vi "CondDoubleArrayProbe.vi"(1 "My Array In":dbl[](array[numeric])) -> (0 "Boolean":bool)   [LabVIEW 2020]
doc: "Monitors an array of double-precision, floating-point numeric controls. The Data tab displays the size of the input array. Use the Conditions tab to set a conditional breakpoint. You can set conditions based on the size of the array or any elements within the array. If you select multiple conditions, LabVIEW executes a breakpoint if any of those conditions are true."
panel:
  in  "Tab Control":enum32{"Data   ", "Conditions      "}(tab)
  out "?":dbl[](array[numeric])
  out "Size of array":i32
  in  "Max Condition":u16(ring) items=["Equal to", "Greater than", "Less than"]
  in  "Max value":dbl
  in  "Maximum value is":bool
  in  "Min Condition":u16(ring) items=["Equal to", "Greater than", "Less than"]
  in  "Min value":dbl
  in  "Minimum value is":bool
  in  "Contains Condition":u16(ring) items=["Equal to", "Greater than", "Less than"]
  in  "Contains value":dbl
  in  "Contains a value":bool
  in  "Number of \nElements Condition":u16(ring) items=["Equal to", "Greater than", "Less than"]
  in  "Number of \nelements value":u32
  in  "Number of \nelements is":bool
  # "Pause if any of the following:"
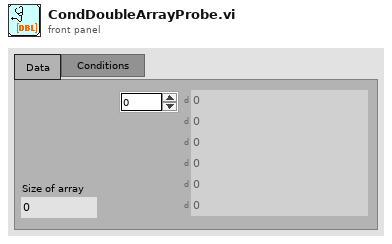
[diagram p1: front panel]
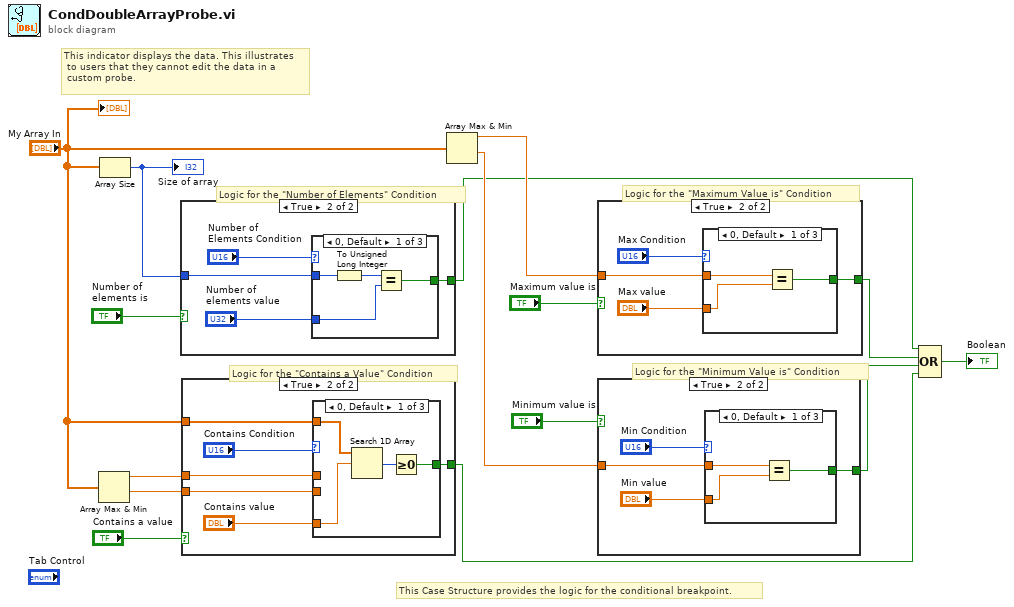
[diagram p0: block diagram]
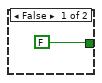
[diagram p2: hidden frame]
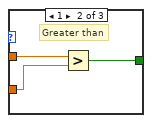
[diagram p3: hidden frame]
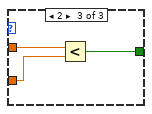
[diagram p4: hidden frame]
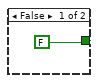
[diagram p5: hidden frame]
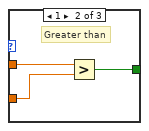
[diagram p6: hidden frame]
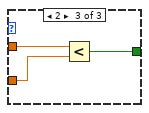
[diagram p7: hidden frame]
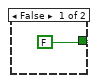
[diagram p8: hidden frame]
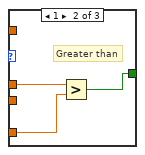
[diagram p9: hidden frame]
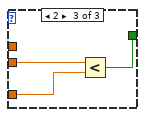
[diagram p10: hidden frame]
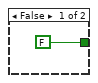
[diagram p11: hidden frame]
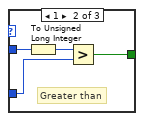
[diagram p12: hidden frame]
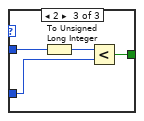
[diagram p13: hidden frame]
diagram:
  # "This indicator displays the data. This illustrates\n to users that they cannot edit the data in a\n custom probe."
  # "Logic for the \"Maximum Value is\" Condition"
  # "Logic for the \"Minimum Value is\" Condition"
  # "Logic for the \"Contains a Value\" Condition"
  # "Logic for the \"Number of Elements\" Condition"
  # "This Case Structure provides the logic for the conditional breakpoint."
  n1 = Array Max & Min(array="My Array In") -> (max value=w12:dbl, min value=w13:dbl)  [unwired: 2 out]
  n2 = Array Size(array="My Array In") -> (size(s)=w14:i32)
  "Size of array" <- w14
  n3 = case shown="True" "Number of \nelements is" {
    tunnel: w14 -> [_ w19]
    tunnel: [FALSE w17] -> w1
    frame False {
    }
    frame True {
      n4 = case shown="0, Default" "Number of \nElements Condition" {
        tunnel: [w24 w26 w30] -> w17
        tunnel: w19 -> [w23 w28 w32]
        tunnel: "Number of \nelements value" -> [w22 w27 w31]
        frame 0, Default {
          n5 = To Unsigned Long Integer(number=w23) -> (unsigned 32bit integer=w21:u32)
          n6 = Equal?(x=w21, y=w22) -> (x = y?=w24:bool)
        }
        frame 1 {
          # "Greater than"
          n7 = To Unsigned Long Integer(number=w28) -> (unsigned 32bit integer=w25:u32)
          n8 = Greater?(x=w25, y=w27) -> (0:w26:bool)
        }
        frame 2 {
          n9 = To Unsigned Long Integer(number=w32) -> (unsigned 32bit integer=w29:u32)
          n10 = Less?(x=w29, y=w31) -> (x < y?=w30:bool)
        }
      }
    }
  }
  n11 = case shown="True" "Contains a value" {
    tunnel: "My Array In" -> [_ w38]
    tunnel: [FALSE w35] -> w5
    tunnel: w12 -> [_ w37]
    tunnel: w13 -> [_ w36]
    frame False {
    }
    frame True {
      n12 = case shown="0, Default" "Contains Condition" {
        tunnel: [w40 w46 w49] -> w35
        tunnel: "Contains value" -> [w42 w44 w48]
        tunnel: w38 -> [w41 _ _]
        tunnel: w37 -> [_ w45 _]
        tunnel: w36 -> [_ _ w47]
        frame 0, Default {
          n13 = Search 1D Array(1D array=w41, element=w42) -> (index of element=w43:i32)  [unwired: 1 in]
          n14 = Greater Or Equal To 0?(x=w43) -> (x >= 0?=w40:bool)
        }
        frame 1 {
          # "Greater than"
          n15 = Greater?(x=w45, y=w44) -> (0:w46:bool)
        }
        frame 2 {
          n16 = Less?(x=w47, y=w48) -> (x < y?=w49:bool)
        }
      }
    }
  }
  n17 = Array Max & Min(array="My Array In") -> (max value=w8:dbl, min value=w7:dbl)  [unwired: 2 out]
  n18 = case shown="True" "Maximum value is" {
    tunnel: [FALSE w52] -> w2
    tunnel: w8 -> [_ w53]
    frame False {
    }
    frame True {
      n19 = case shown="0, Default" "Max Condition" {
        tunnel: [w57 w58 w61] -> w52
        tunnel: w53 -> [w56 w60 w63]
        tunnel: "Max value" -> [w55 w59 w62]
        frame 0, Default {
          n20 = Equal?(x=w56, y=w55) -> (x = y?=w57:bool)
        }
        frame 1 {
          # "Greater than"
          n21 = Greater?(x=w60, y=w59) -> (0:w58:bool)
        }
        frame 2 {
          n22 = Less?(x=w63, y=w62) -> (x < y?=w61:bool)
        }
      }
    }
  }
  n23 = case shown="True" "Minimum value is" {
    tunnel: w7 -> [_ w66]
    tunnel: [FALSE w65] -> w3
    frame False {
    }
    frame True {
      n24 = case shown="0, Default" "Min Condition" {
        tunnel: [w71 w72 w75] -> w65
        tunnel: w66 -> [w70 w74 w77]
        tunnel: "Min value" -> [w69 w73 w76]
        frame 0, Default {
          n25 = Equal?(x=w70, y=w69) -> (x = y?=w71:bool)
        }
        frame 1 {
          # "Greater than"
          n26 = Greater?(x=w74, y=w73) -> (0:w72:bool)
        }
        frame 2 {
          n27 = Less?(x=w77, y=w76) -> (x < y?=w75:bool)
        }
      }
    }
  }
  n28 = Compound Arithmetic op=OR(w1, w2, w3, w5) -> (→"Boolean":bool)
  "?" <- "My Array In"
